vi "SegmentParamsDialog.vi"() -> ()   [LabVIEW 2012]
panel:
  in  "MaxRateText":dbl caption="°C/My"
  in  "Cancel Button":bool
  in  "OK Button":bool
  in  "MaxRate":bool caption="Impose maximum dT/dt:"
  in  "Randomizer":string(combo) caption="Randomizer style:"
  in  "SegDivs":string(combo) caption="Halve:"
  in  "SegType":string(combo) caption="Path between constraints:"
  # "times"
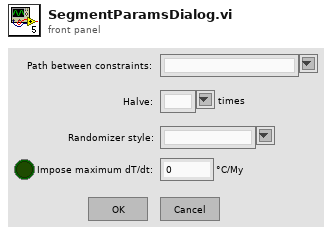
[diagram p1: front panel]
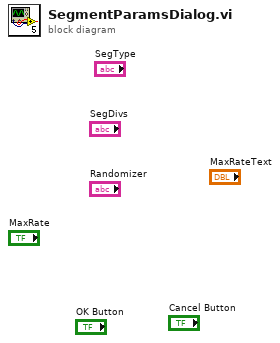
[diagram p0: block diagram]
diagram:
